vi "Collect_Beam_Positions.vi"(1 "Align Probe Using":enum16{"Green Beams", "Blue Beams"}(ring), 2 "Use Specification Beam Half-Angle":bool) -> ()   [LabVIEW 2011]
uses:
  Controls/Tunnel_Coordinates.ctl
  Controls/User_Specific_mode.ctl
  Gen Trav/Trav_mode.ctl
  Globals/Trav_pos_global.vi
  Globals/Constants_global.vi
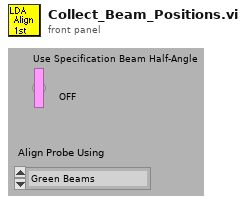
[diagram p1: front panel]
types:
  T1 = typedef "Tunnel_Coordinates.ctl" = enum16{"Work in Tunnel Coordinates", "Work in Model Coordinates"}
  T2 = typedef "User_Specific_mode.ctl" = enum16{"Check VI only", "Run VI"}
  T3 = typedef "Trav_mode.ctl" = enum16{"Move traverse", "Read traverse position", "Teach Position"}
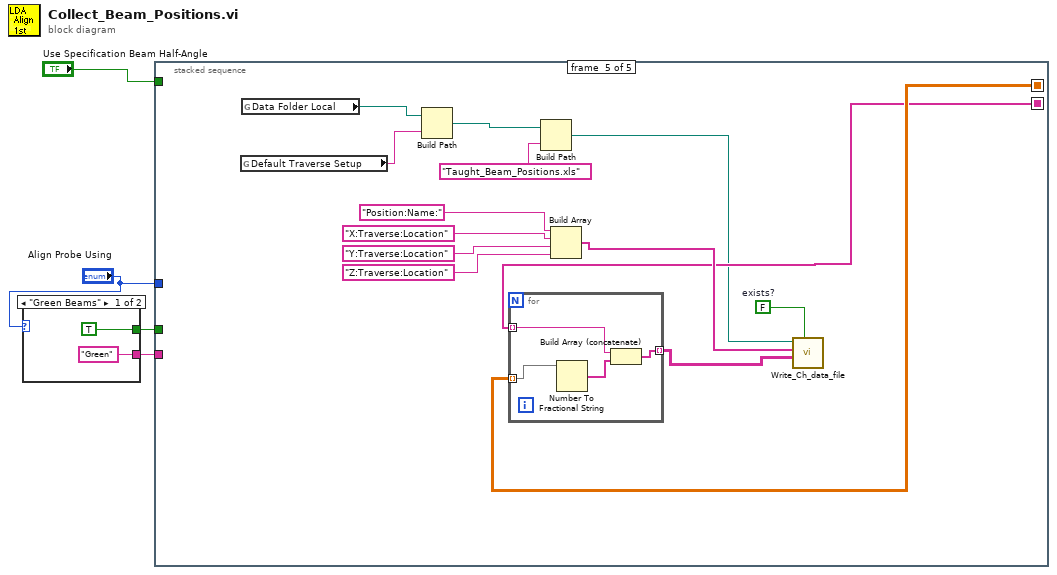
[diagram p0: block diagram]
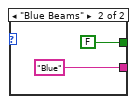
[diagram p2: hidden frame]
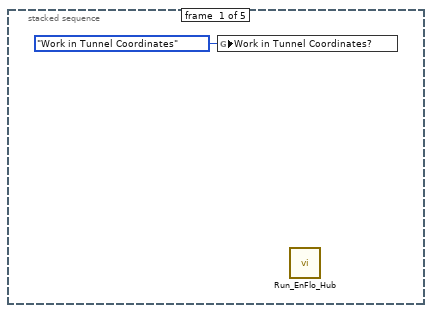
[diagram p3: hidden frame]
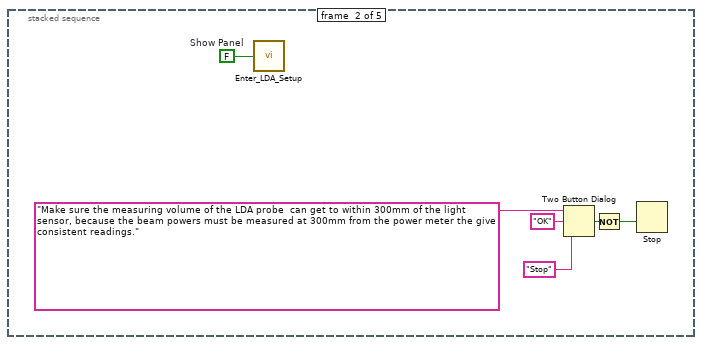
[diagram p4: hidden frame]
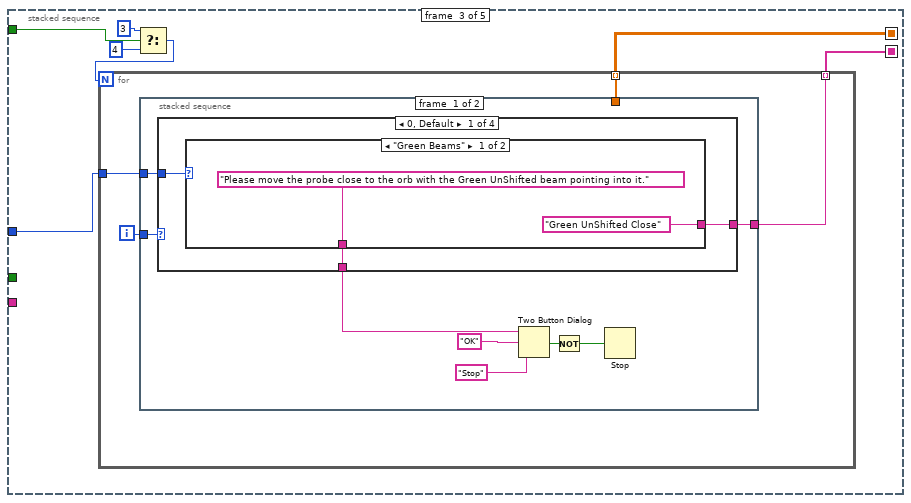
[diagram p5: hidden frame]
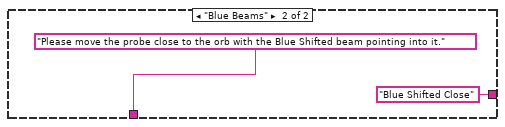
[diagram p6: hidden frame]
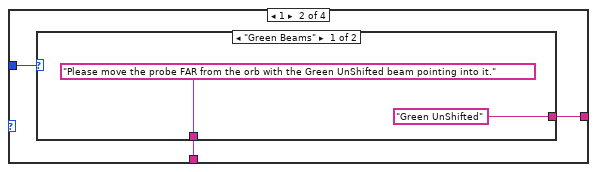
[diagram p7: hidden frame]
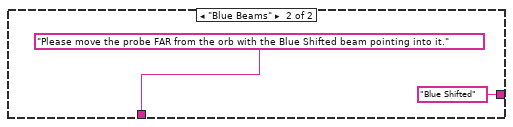
[diagram p8: hidden frame]
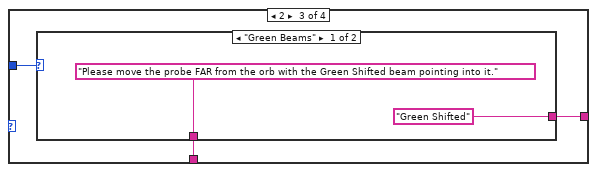
[diagram p9: hidden frame]
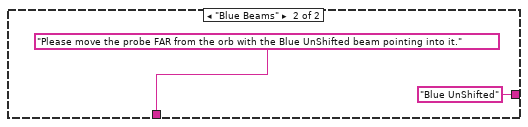
[diagram p10: hidden frame]
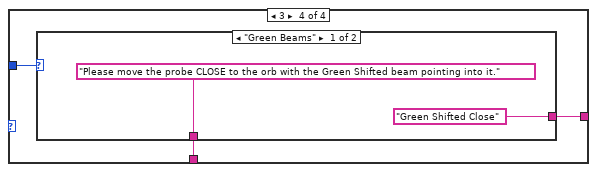
[diagram p11: hidden frame]
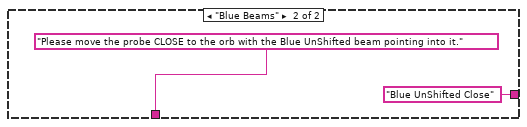
[diagram p12: hidden frame]
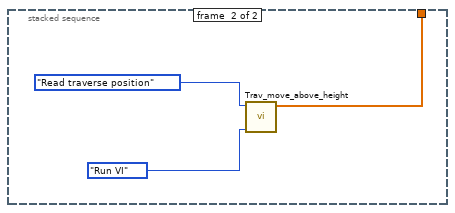
[diagram p13: hidden frame]
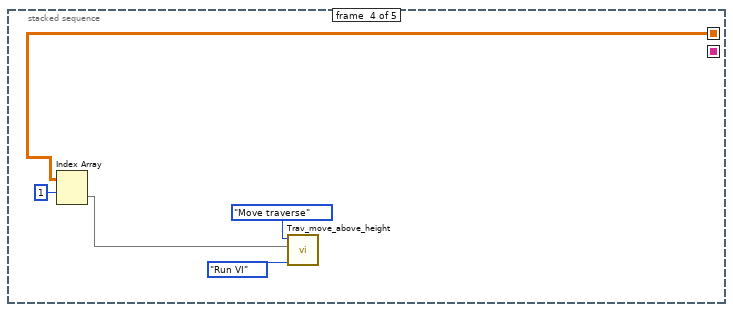
[diagram p14: hidden frame]
diagram:
  n1 = case shown="\"Green Beams\"" "Align Probe Using" {
    tunnel: [TRUE FALSE] -> w4
    tunnel: ["Green" "Blue"] -> w1
    frame "Green Beams" {
    }
    frame "Blue Beams" {
    }
  }
  n2 = stacked-sequence {
    seq-local: [_ _ w17 _ _] -> [_ _ _ w68 w74]
    seq-local: [_ _ w16 _ _] -> [_ _ _ _ w73]
    tunnel: w4 -> [_ _ _ _ _]
    tunnel: "Use Specification Beam Half-Angle" -> [_ _ w21 _ _]
    tunnel: "Align Probe Using" -> [_ _ w22 _ _]
    tunnel: w1 -> [_ _ _ _ _]
    frame #0 {
      n3 = global write "Trav_pos_global.vi" "Work in Tunnel Coordinates?"(Tunnel_Coordinates."Work in Tunnel Coordinates" ("Work in Tunnel Coordinates?")) -> ()
      n4 = call "Run_EnFlo_Hub.vi"() -> ()  [unwired: 8 out]
    }
    frame #1 {
      w15 = FALSE  # Show Panel
      n5 = call "Enter_LDA_Setup.vi"("Show Panel"=w15) -> ()
      n6 = Two Button Dialog(message="Make sure the measuring volume of the LDA probe  can get to within 300mm of the light sensor, because the beam powers must be measured at 300mm from the power meter the give consistent readings.", 1:"Stop" ("F button name (\"Cancel\")"), 2:"OK" ("T button name (\"OK\")")) -> (T button?=w11:bool)
      n7 = Not(x=w11) -> (.not. x?=w10:bool)
      n8 = Stop(stop? (T)=w10) -> ()
    }
    frame #2 {
      n9 = Select(t=3, s=w21, f=4) -> (s? t:f=w18:i32)
      n10 = for {
        N: w18 -> [_]
        tunnel: [w26] -> w17 mode=indexing
        tunnel: w22 -> [w25]
        tunnel: [w24] -> w16 mode=indexing
        i -> [w23]
        n11 = stacked-sequence {
          tunnel: [_ w63] -> w26
          tunnel: w25 -> [w33 _]
          tunnel: [w28 _] -> w24
          tunnel: w23 -> [w27 _]
          frame #0 {
            n12 = case shown="0, Default" w27 {
              tunnel: [w37 w44 w51 w58] -> w34
              tunnel: w33 -> [w36 w43 w50 w57]
              tunnel: [w35 w42 w49 w56] -> w28
              frame 0, Default {
                n13 = case shown="\"Green Beams\"" w36 {
                  tunnel: ["Please move the probe close to the orb with the Green UnShifted beam pointing into it." ("message") "Please move the probe close to the orb with the Blue Shifted beam pointing into it." ("message")] -> w37
                  tunnel: ["Green UnShifted Close" "Blue Shifted Close"] -> w35
                  frame "Green Beams" {
                  }
                  frame "Blue Beams" {
                  }
                }
              }
              frame 1 {
                n14 = case shown="\"Green Beams\"" w43 {
                  tunnel: ["Please move the probe FAR from the orb with the Green UnShifted beam pointing into it." ("message") "Please move the probe FAR from the orb with the Blue Shifted beam pointing into it." ("message")] -> w44
                  tunnel: ["Green UnShifted" "Blue Shifted"] -> w42
                  frame "Green Beams" {
                  }
                  frame "Blue Beams" {
                  }
                }
              }
              frame 2 {
                n15 = case shown="\"Green Beams\"" w50 {
                  tunnel: ["Please move the probe FAR from the orb with the Green Shifted beam pointing into it." ("message") "Please move the probe FAR from the orb with the Blue UnShifted beam pointing into it." ("message")] -> w51
                  tunnel: ["Green Shifted" "Blue UnShifted"] -> w49
                  frame "Green Beams" {
                  }
                  frame "Blue Beams" {
                  }
                }
              }
              frame 3 {
                n16 = case shown="\"Green Beams\"" w57 {
                  tunnel: ["Please move the probe CLOSE to the orb with the Green Shifted beam pointing into it." ("message") "Please move the probe CLOSE to the orb with the Blue UnShifted beam pointing into it." ("message")] -> w58
                  tunnel: ["Green Shifted Close" "Blue UnShifted Close"] -> w56
                  frame "Green Beams" {
                  }
                  frame "Blue Beams" {
                  }
                }
              }
            }
            n17 = Two Button Dialog(message=w34, 1:"Stop" ("F button name (\"Cancel\")"), 2:"OK" ("T button name (\"OK\")")) -> (T button?=w30:bool)
            n18 = Not(x=w30) -> (.not. x?=w29:bool)
            n19 = Stop(stop? (T)=w29) -> ()
          }
          frame #1 {
            n20 = call "Trav_move_above_height.vi"("Simulate/Run"=User_Specific_mode."Run VI", "Mode"=Trav_mode."Read traverse position") -> ("Trav Position achieved"=w63:dbl[])  [unwired: 5 in, 4 out]
          }
        }
      }
    }
    frame #3 {
      n21 = Index Array(array=w68, index (row)=1) -> (element=w66:dbl[])  [unwired: 1 in]
      n22 = call "Trav_move_above_height.vi"("Simulate/Run"=User_Specific_mode."Run VI", "New Position"=w66, "Mode"=Trav_mode."Move traverse") -> ()  [unwired: 4 in, 5 out]
    }
    frame #4 {
      w76 = FALSE  # exists?
      n23 = global read "Trav_pos_global.vi" "Default Traverse Setup"() -> (w83:string)
      n24 = global read "Constants_global.vi" "Data Folder Local"() -> (w81:path)
      n25 = Build Path(base path=w81, name or relative path=w83) -> (appended path=w82:path)
      n26 = for {
        tunnel: w74 -> [w88] mode=indexing
        tunnel: w73 -> [w87] mode=indexing
        tunnel: [w85] -> w72 mode=indexing
        n27 = Number To Fractional String(number=w88) -> (F-format string=w86:string[])  [unwired: 3 out]
        n28 = Build Array (concatenate)(w87, w86) -> (w85:string[])
      }
      n29 = Build Path(base path=w82, name or relative path="Taught_Beam_Positions.xls" ("Substring")) -> (appended path=w71:path)
      n30 = Build Array("Position:Name:", "X:Traverse:Location", "Y:Traverse:Location", "Z:Traverse:Location") -> (w75:string[])
      n31 = call "Write_Ch_data_file.vi"("exists?"=w76, "Channel Values"=w72, "Channel names"=w75, "Filename"=w71) -> ()  [unwired: 4 in, 4 out]
    }
  }
